vi "SetUpHelper.vi"(8 "ErrorIn":errorcluster, 11 "Reference":T1) -> (0 "ErrorOut":errorcluster, 3 "OutConnection":T1)   [LabVIEW 2019]
uses:
  C:/Users/yasav/Downloads/prev_robocad/robocadSimLVFolder/assemblies/LibraryForLabVIEW.dll
  assemblies/LibraryForLabVIEW.dll
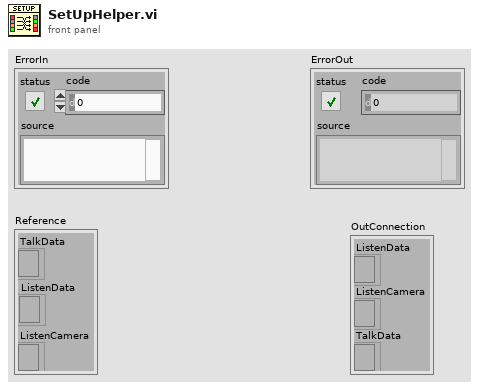
[diagram p1: front panel]
types:
  T1 = cluster{"ListenData":refnum<k24>, "ListenCamera":refnum<k24>, "TalkData":refnum<k24>}
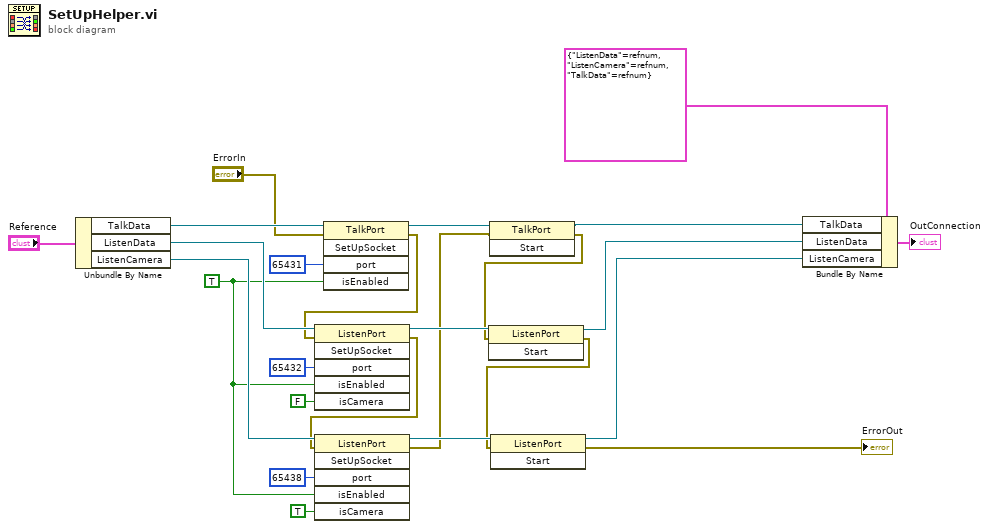
[diagram p0: block diagram]
diagram:
  w7 = TRUE
  n1 = Unbundle By Name("Reference") -> ("TalkData"=w10:refnum<k24>, "ListenData"=w22:refnum<k24>, "ListenCamera"=w19:refnum<k24>)
  n2 = invoke class="TalkPort" method="SetUpSocket"(reference=w10, error in="ErrorIn", "port"=65431, "isEnabled"=w7) -> (reference out=w6:refnum<k24>, error out=w8:errorcluster)  [unwired: 1 in, 3 out]
  n3 = invoke class="ListenPort" method="SetUpSocket"(reference=w22, error in=w8, "port"=65432, "isEnabled"=w7, "isCamera"=FALSE) -> (reference out=w17:refnum<k24>, error out=w18:errorcluster)  [unwired: 1 in, 4 out]
  n4 = invoke class="ListenPort" method="SetUpSocket"(reference=w19, error in=w18, "port"=65438, "isEnabled"=w7, "isCamera"=TRUE) -> (reference out=w16:refnum<k24>, error out=w3:errorcluster)  [unwired: 1 in, 4 out]
  n5 = invoke class="TalkPort" method="Start"(reference=w6, error in=w3) -> (reference out=w5:refnum<k24>, error out=w4:errorcluster)  [unwired: 1 in, 1 out]
  n6 = invoke class="ListenPort" method="Start"(reference=w17, error in=w4) -> (reference out=w13:refnum<k24>, error out=w15:errorcluster)  [unwired: 1 in, 1 out]
  n7 = invoke class="ListenPort" method="Start"(reference=w16, error in=w15) -> (reference out=w12:refnum<k24>, error out=→"ErrorOut":errorcluster)  [unwired: 1 in, 1 out]
  n8 = Bundle By Name(cluster=T1 {"ListenData"=refnum, "ListenCamera"=refnum, "TalkData"=refnum}, "TalkData"=w5, "ListenData"=w13, "ListenCamera"=w12) -> (→"OutConnection":T1)
